vi "Dashboard Main 2022.vi"(0 "Dashboard Tab":T3(tab)) -> ()   [LabVIEW 2020]
uses:
  <vilib>/Rock Robotics/Network Tables/NT Read Number.vi
  <vilib>/Rock Robotics/Network Tables/NT Read Numeric Array.vi
  <vilib>/Rock Robotics/Network Tables/NT Read String.vi
  <vilib>/Rock Robotics/Network Tables/NT Read Boolean.vi
  <vilib>/Rock Robotics/Network Tables/NT Write Number.vi
  <vilib>/Rock Robotics/Network Tables/NT Write Boolean.vi
panel:
  out "Robot IP":string
  out "Popcorn Engaged":bool
  out "Camera Image 5":T1(plugin-control)
  out "Camera Perf":string
  in  "Camera Settings":T2={"Frame Rate"=30, "Compression"=30, "Size"=1, "DB Camera Config"=FALSE} {"Frame Rate" scale=1.0..30.0; "Compression" scale=100.0..-1.0; "Size" items=["640x480", "320x240", "160x120"]}
  in  "TCP":refnum<k5>
  out "MotorChart R":cluster{"Numeric":dbl, "Numeric":dbl}(graph)
  out "MotorChart L":cluster{"Numeric":dbl, "Numeric":dbl}(graph)
  out "MotorSliders R":cluster{"MotorSlide1":dbl, "MotorSlide2":dbl} {"MotorSlide2" scale=-1.0..1.0 scale format="%#_2e"; "MotorSlide1" scale=-1.0..1.0 scale format="%#_2e"}
  out "MotorSliders L":cluster{"MotorSlide1":dbl, "MotorSlide2":dbl} {"MotorSlide2" scale=-1.0..1.0 scale format="%#_2e"; "MotorSlide1" scale=-1.0..1.0 scale format="%#_2e"}
  out "To infinity and beyond?":string
  out "Climb Override":bool
  out "Climbing Stages":sgl(slide) scale=0.0..10.0 scale format="%#_6p"
  out "Reverse":bool
  in  "ARE YOU READY TO RUMBLE":bool
  out "Drive Mode":string
  in  "Select Auto":string(combo)="Select Autonomous ..."
  out "NT Connection":bool
  out "JS1 Z":dbl(slide) scale=-1.0..1.0 scale format="%#_2e"
  out "JS1 Graph":cluster{"X":dbl, "Y":dbl}[](graph)
  out "JS1 Buttons":T4
  out "JS2 Z":dbl(slide) scale=-1.0..1.0 scale format="%#_2e"
  out "JS2 Graph":cluster{"X":dbl, "Y":dbl}[](graph)
  out "JS2 Buttons":T4
  out "Lidar":dbl(knob) scale=0.0..10.0
  out "Wall!":bool
  out "Mode":T5(ring)=enum."Auto Disabled"
  out "Motor Output":dbl
  out "Target Shooter Speed":dbl
  out "Shooter Speed":T6(graph)
  out "Shooter Speed":dbl
  in  "Shooter Demand":dbl
  in  "Dashboard Tab 2":T7(tab)
  out "Speed Chart Left":cluster{"Numeric":dbl, "Numeric":dbl}(graph)
  out "Speed Chart Right":cluster{"Numeric":dbl, "Numeric":dbl}(graph)
  in  "Dont Question it":bool
  out "Right Speed Demand":dbl
  out "Left Speed Demand":dbl
  out "Right Speed":dbl
  out "Left Speed":dbl
  out "Deviation Threshold":dbl
  out "Filter Height":dbl
  in  "Deviation Threshold":dbl
  in  "Filter Height":dbl
  out "Current Filter":T8={"Hue"={110.0, 142.0}, "Saturation"={0.0, 209.6394230769231}, "Value"={0.0, 105.16949152542372}} {"Value" scale=0.0..255.0; "Saturation" scale=0.0..255.0; "Hue" scale=0.0..255.0 scale format="%#_3g"}
  in  "New Filter":T8={"Hue"={110.0, 142.0}, "Saturation"={0.0, 209.6394230769231}, "Value"={0.0, 105.16949152542372}} {"Value" scale=0.0..255.0; "Saturation" scale=0.0..255.0; "Hue" scale=0.0..255.0 scale format="%#_3g"}
  out "Bananas Engaged":bool
  in  "DONUT PRESS":bool
  out "Bandwidth (Mbps)":dbl
  out "FPS":dbl
  in  "Update":bool
  in  "CheckList":i32[](listbox)
  out "Tree":string(tree)
  out "Camera Image":T1(plugin-control)
  out "Background":bool
  in  "Camera Name":string(combo)="No Camera Selection"
  # "HW"
  # "Joysticks"
  # "Drive Motors"
  # "Front"
  # "Right"
  # "Left"
  # "Back"
  # "Right"
  # "Left"
  # "Speed D"
  # "Speed"
  # "DONUT PRESS"
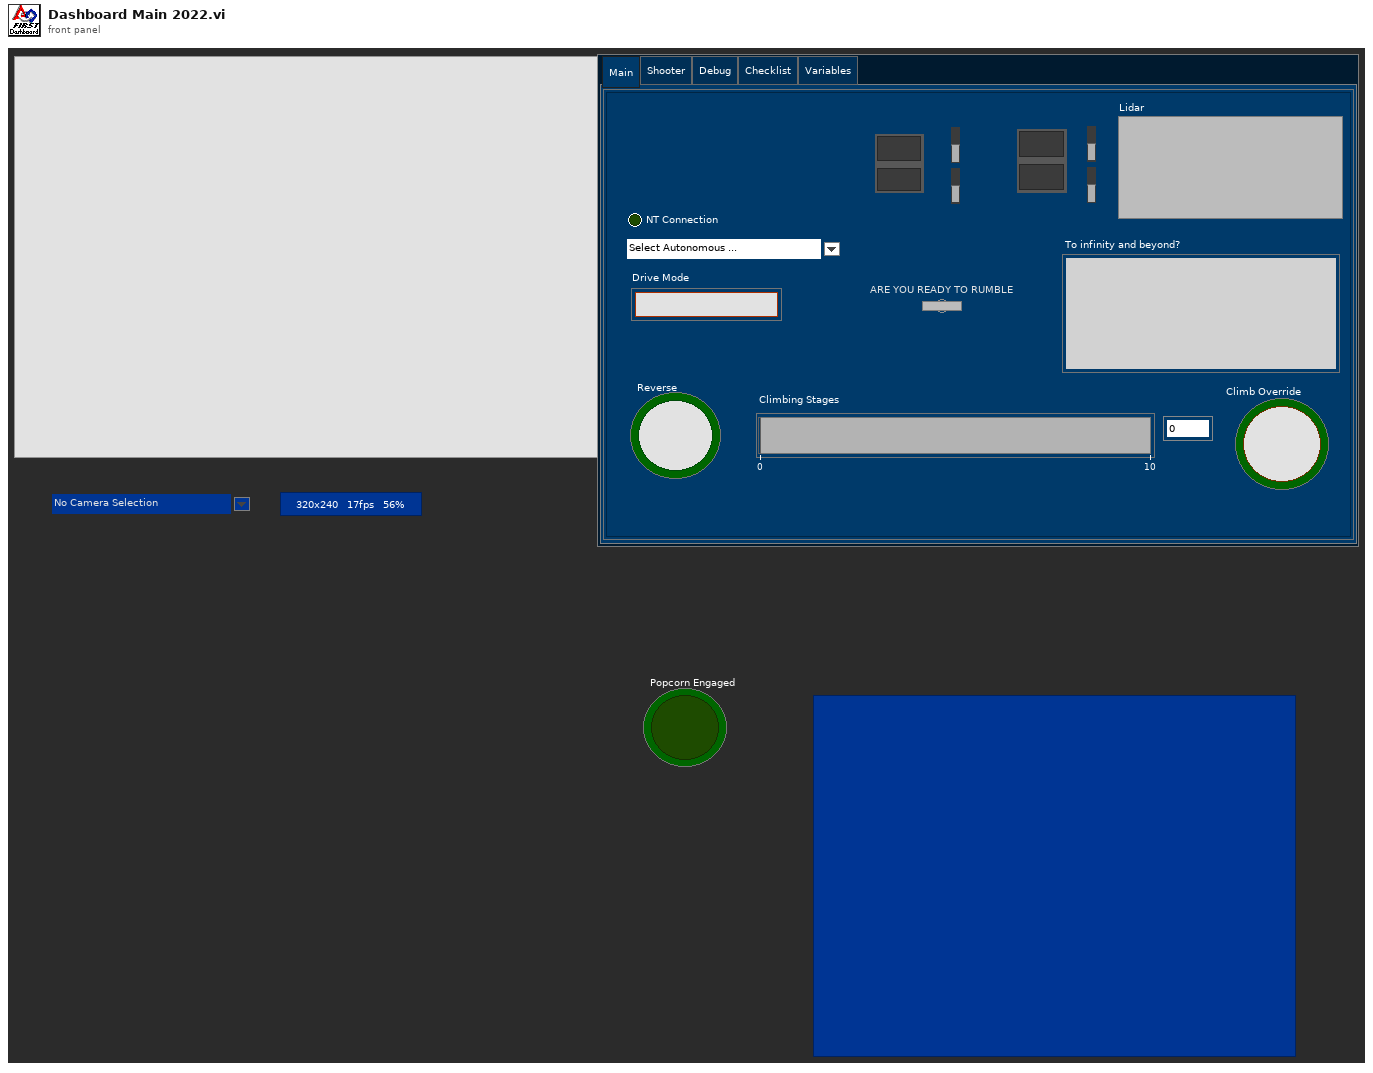
[diagram p1: front panel]
types:
  T1 = typedef "IMAQ Image.ctl" = refnum<image>
  T2 = cluster{"Frame Rate":i32, "Compression":i32, "Size":u16, "DB Camera Config":bool}
  T3 = enum32{"Main", "Shooter", "Debug", "Checklist", "Variables"}
  T4 = cluster{bool, bool, bool, bool, bool, bool, bool, bool, bool, bool, bool, bool}
  T5 = enum8{"Tele-Op Disabled", "Tele-Op Enabled", "Auto Disabled", "Auto Enabled", "Test Disabled", "Test Enabled", "Disconnected", "No Code", "E-Stop"}
  T6 = cluster{"Shooter Demand":dbl, "Numeric":dbl, "Numeric":dbl}
  T7 = enum32{"Drive Left", "Drive Right", "Table", "Camera", "Random"}
  T8 = cluster{"Hue":cluster{dbl, dbl}, "Saturation":cluster{dbl, dbl}, "Value":cluster{dbl, dbl}}
  T9 = cluster{"Save Path":path, "Interval (s)":dbl, "Keep":i32}
  T10 = typedef "Image Type" = u32
  T11 = cluster{"Camera Image":refnum<vi>, "Dashboard Tab":refnum<vi>, "Background":refnum<vi>, "Tree":refnum<vi>, "Camera Settings":refnum<vi>, "Camera Name":refnum<vi>, "Camera Perf":refnum<vi>}
  T12 = cluster{"Camera Name":string, "Camera File Name":string, "Saved DB Images Info":cluster{"Save Path":path, "Interval (s)":dbl, "Keep":i32}}
  T13 = cluster{cluster{dbl, dbl}, cluster{dbl, dbl}, cluster{dbl, dbl}}
  T14 = cluster{"Shift":bool, "Ctrl":bool, "Alt":bool, "Cmd":bool, "Opt":bool}
  T15 = cluster{"Error Strings":string, "Disable Counts":cluster{u16, u16}, "Rail Faults":cluster{u16, u16, u16}, "Robot IP":string, "DB Mode":u8, "Event Info":cluster{"Name":string, "Type":u8, "Number":u16, "Replay":u8}}
  T16 = cluster{"Storage":cluster{"Disk Free":u64, "RAM Block":u32, "RAM free":u32}, "CPU Utilization":cluster{"CPU % ISR":sgl, "CPU % Time Crit":sgl, "CPU % Timed Str":sgl, "CPU % High":sgl, "CPU % Above":sgl, "CPU % Normal":sgl, "CPU % Low":sgl}, "CAN":cluster{"% Bus Utilization":sgl, "Bus Off Cnt":u32, "TX_FIFO Full Cnt":u32, "Receive Error Cnt":u8, "Transmit Error Cnt":u8}, "HID":cluster{"HID Outputs":u32, "Rumble Low":u16, "Rumble High":u16}[]}
  T17 = cluster{"Status bits":cluster{"Test Mode":bool, "Autonomous":bool, "Enabled":bool, "Code Start":bool, "Brownout":bool, "Reserved 2":bool, "Reserved 3":bool, "E-Stop":bool}, "Code Trace":cluster{"Disabled":bool, "TeleOp":bool, "Auto":bool, "Test":bool}, "Controller Type":enum16{"unknown", "cRIO", "roboRio"}, "Code?":enum16{"unknown", "noCode", "code"}, "Battery V":dbl}
  T18 = cluster{"Control Bits":cluster{"TestMode":bool, "Autonomous":bool, "Enabled":bool, "FMS Present":bool, bool, bool, bool, "E-Stop":bool}, "Team Station ":u8, "Countdown":sgl, "Joystick Values":cluster{"Axes":dbl[], "Buttons":bool[], "POVs":i16[]}[]}
  T19 = cluster{"Axes":dbl[], "Buttons":bool[], "POVs":i16[]}[]
  T20 = cluster{"Axes":dbl[], "Buttons":bool[], "POVs":i16[]}
  T21 = cluster{"Buttons[0]":bool, "Buttons[1]":bool, "Buttons[2]":bool, "Buttons[3]":bool, "Buttons[4]":bool, "Buttons[5]":bool, "Buttons[6]":bool, "Buttons[7]":bool, "Buttons[8]":bool, "Buttons[9]":bool, "Buttons[10]":bool, "Buttons[11]":bool}
  T22 = cluster{"Shooter Demand":dbl, "value":dbl, "value":dbl}
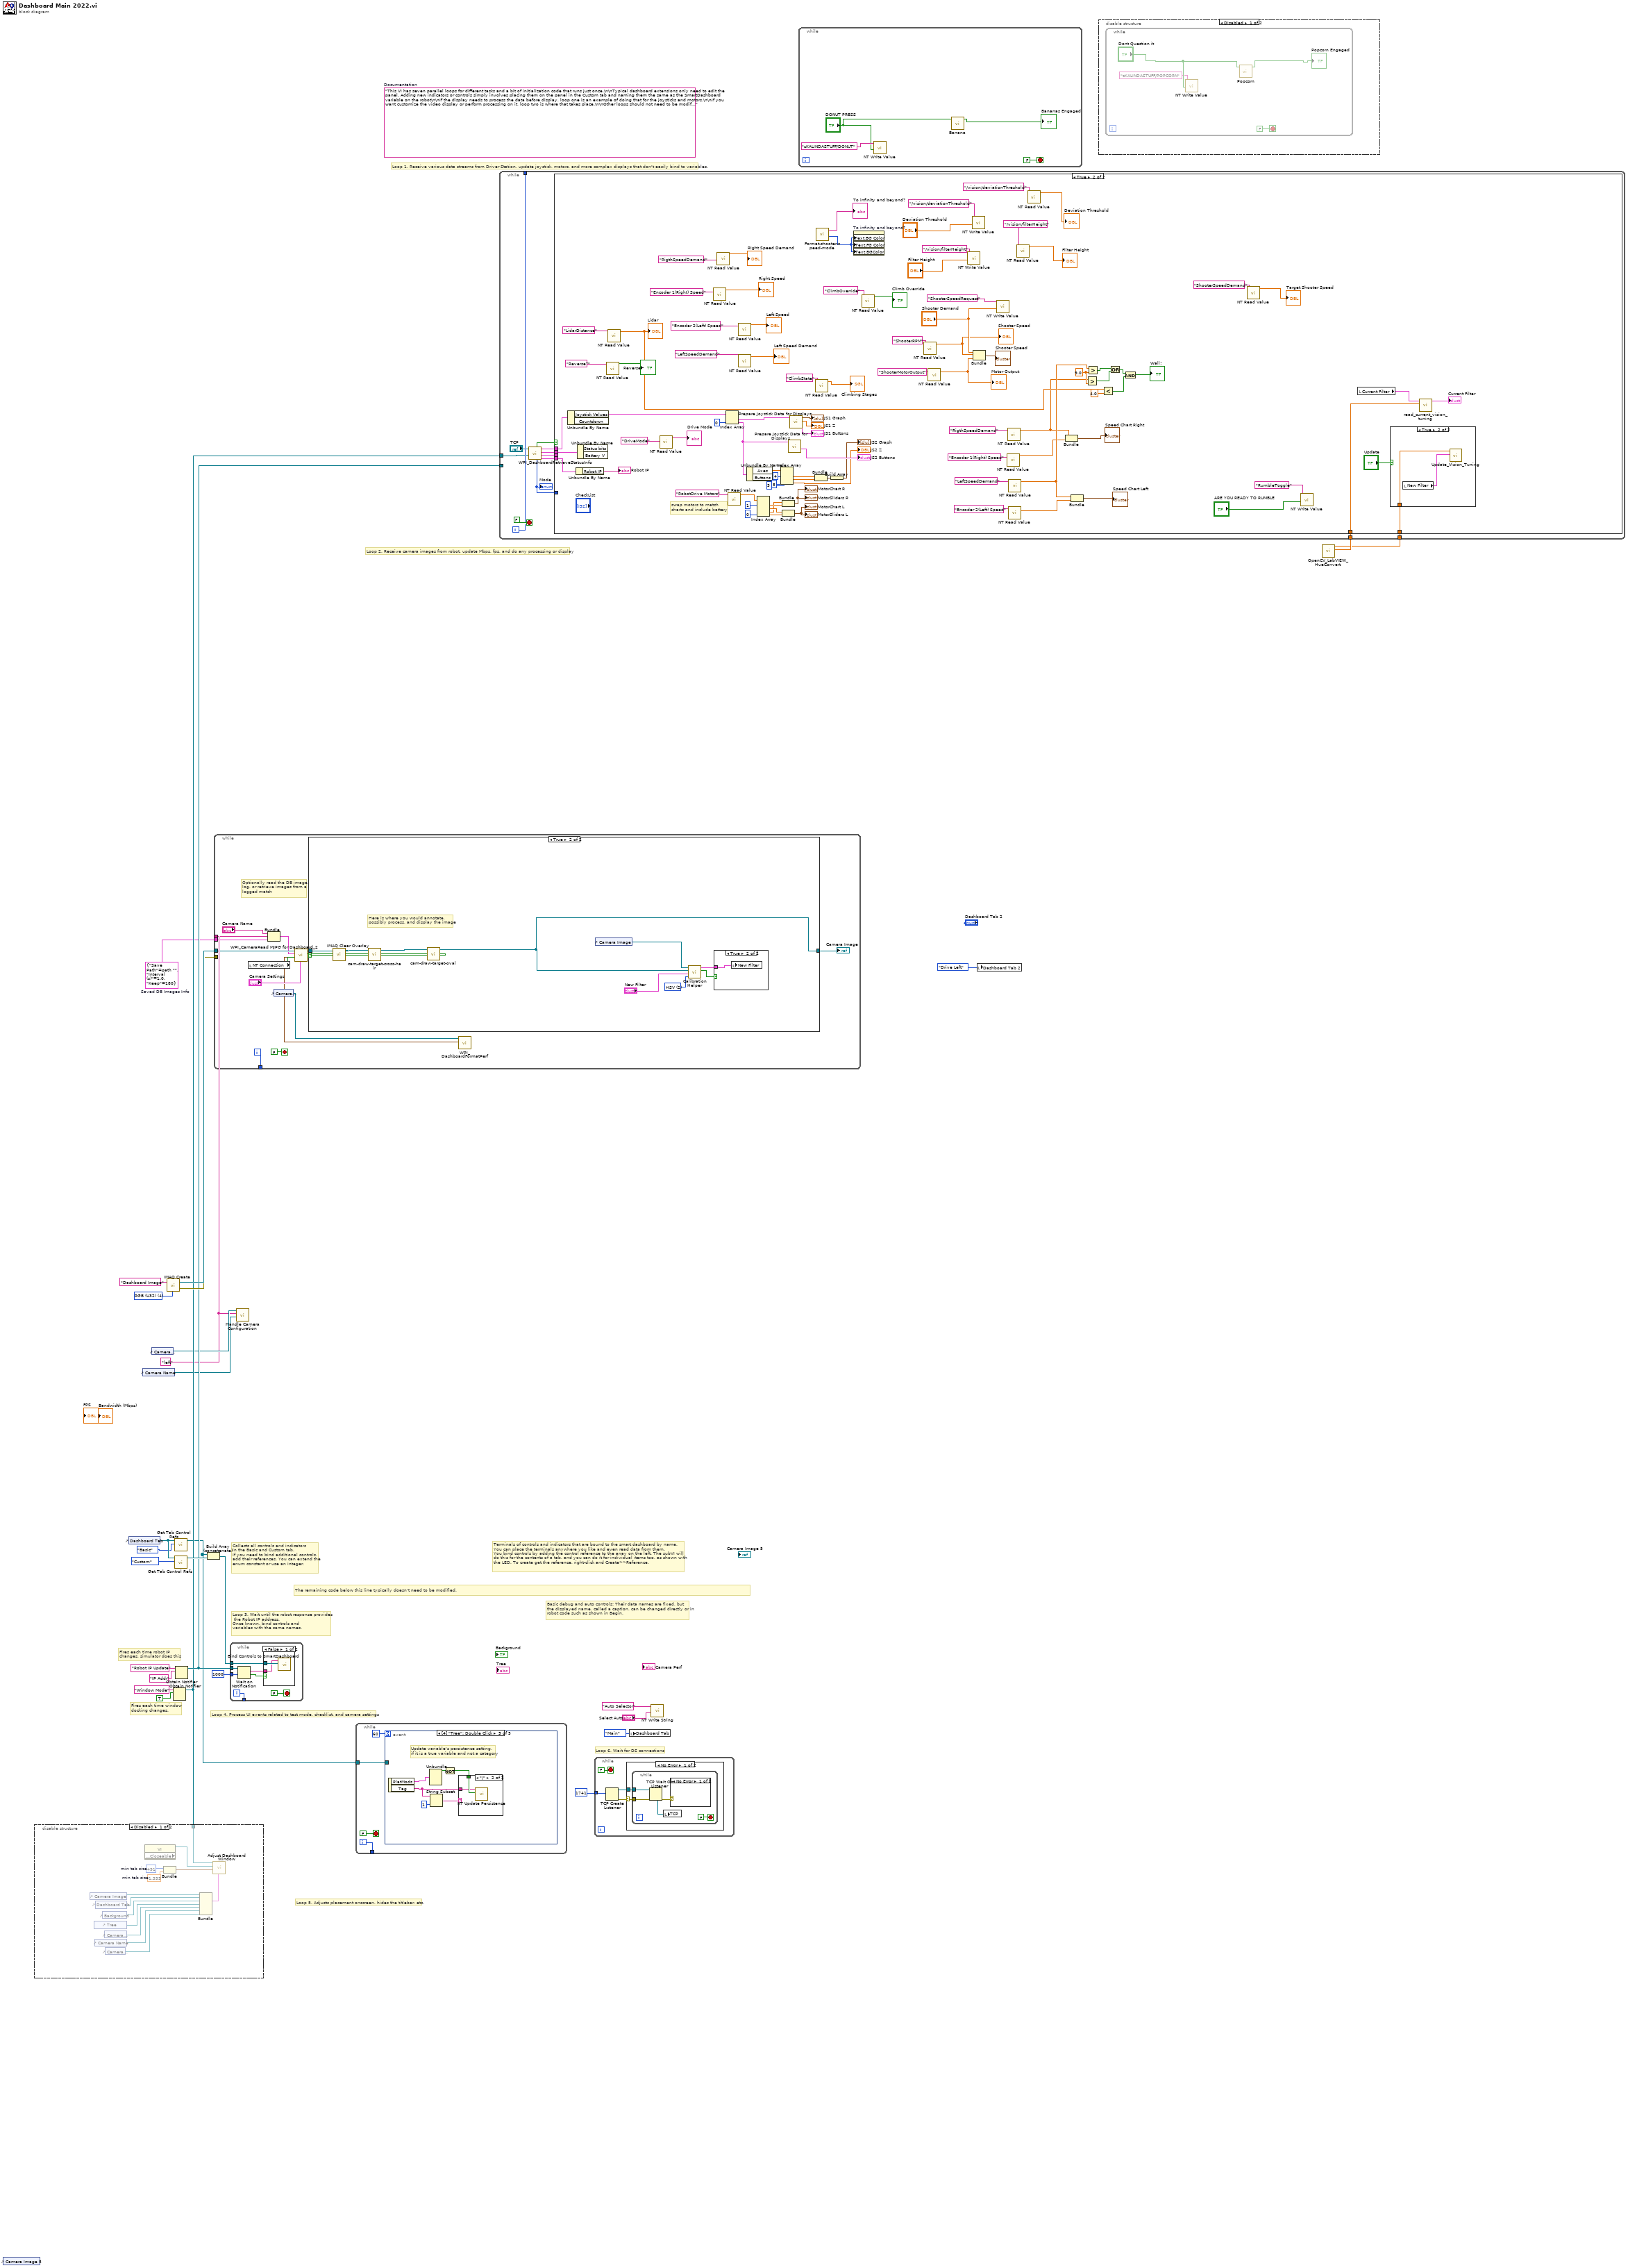
[diagram p0: block diagram]
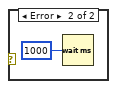
[diagram p4: hidden frame]
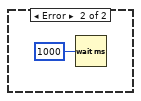
[diagram p5: hidden frame]
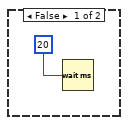
[diagram p6: hidden frame]
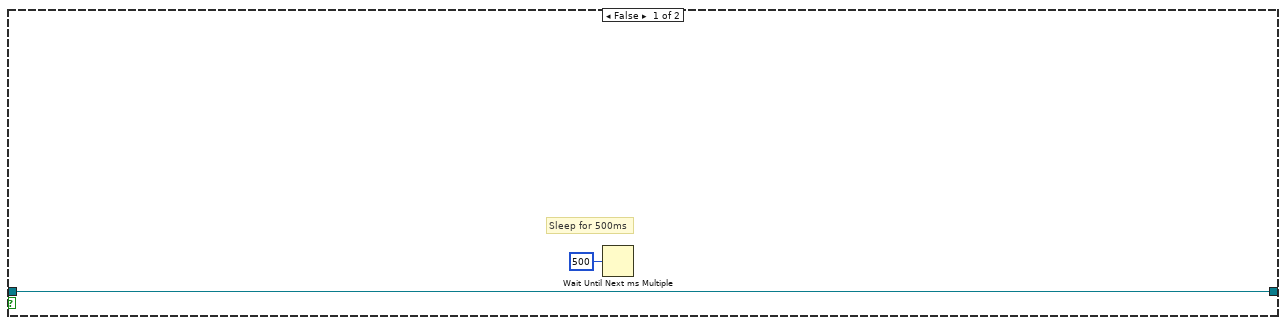
[diagram p9: hidden frame]
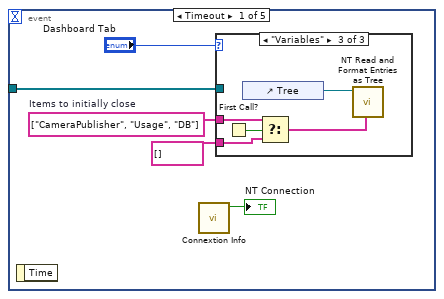
[diagram p11: hidden frame]
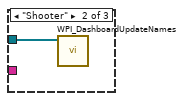
[diagram p13: hidden frame]
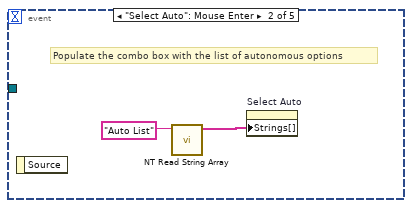
[diagram p14: hidden frame]
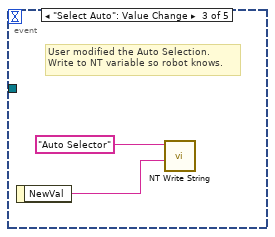
[diagram p15: hidden frame]
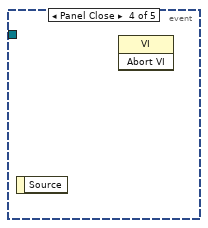
[diagram p16: hidden frame]
diagram:
  w6 = "left" ("Camera File Name")
  w5 = T9 {"Save Path"=path "", "Interval (s)"=1.0, "Keep"=180}  # Saved DB Images Info
  (unwired) "This VI has seven parallel loops for different tasks and a bit of initialization code that runs just once.\n\nTypical dashboard extensions only need to edit the panel. Adding new indicators or controls simply involves placing them on the panel in the Custom tab and naming them the same as the SmartDashboard variable on the robot\n\nIf the display needs to process the data before display, loop one is an example of doing that for the joysticks and motors.\n\nIf you want customize the video display or perform processing on it, loop two is where that takes place.\n\nOther loops should not need to be modified. They are pretty standard, and document the task they perform."  # Documentation
  w28 = T10 4 items=["Grayscale (U8)", "Grayscale (I16)", "Grayscale (SGL)", "Complex (CSG)", "RGB (U32)", "HSL (U32)", "RGB (U64)"] ("Image Type")
  # "Loop 5. Adjusts placement onscreen, hides the titlebar, etc."
  # "Loop 6. Wait for DS connections"
  # "Basic debug and auto controls: Their data names are fixed, but\nthe displayed name, called a caption, can be changed directly or in\nrobot code such as shown in Begin."
  # "Fires each time robot IP\nchanges, simulator does this"
  # "Fires each time window\ndocking changes."
  # "Collects all controls and indicators\nin the Basic and Custom tab.\nIf you need to bind additional controls,\nadd their references. You can extend the\nenum constant or use an integer."
  # "The remaining code below this line typically doesn't need to be modified."
  # "Loop 4. Process UI events related to test mode, checklist, and camera settings"
  # "Terminals of controls and indicators that are bound to the smart dashboard by name.\nYou can place the terminals anywhere you like and even read data from them.\nYou bind controls by adding the control reference to the array on the left. The subVI will\ndo this for the contents of a tab, and you can do it for individual items too, as shown with\nthe LED. To create get the reference, right-click and Create>>Reference."
  # "Loop 3. Wait until the robot response provides\n the Robot IP address.\nOnce known, bind controls and\nvariables with the same names."
  # "Loop 1. Receive various data streams from Driver Station, update joystick, motors, and more complex displays that don't easily bind to variables."
  # "Loop 2. Receive camera images from robot, update Mbps, fps, and do any processing or display"
  n1 = control-ref of="Camera Image 5"() -> ()  [unwired: 1 out]
  n2 = control-ref of="Dashboard Tab"() -> (w19:refnum<vi>)
  n3 = control-ref of="Camera Name"() -> (w12:refnum<vi>)
  n4 = control-ref of="Camera Settings"() -> (w13:refnum<vi>)
  n5 = call "IMAQ Create"("Image Name"="Dashboard Image", "Image Type"=w28) -> ("New Image"=w26:T1, "error out"=w25:errorcluster)  [unwired: 2 in, 1 out]
  n6 = Obtain Notifier(name (unnamed)="Window Mode", notification data type=TRUE) -> (notifier out=w15:refnum<notifier>)  [unwired: 2 in, 2 out]
  n7 = disable-structure shown="Disabled" {
    disable-tunnel: w15 -> [w33 _]
    frame Disabled {
      w38 = 491  # min tab size
      w37 = 1.333  # min tab size
      n8 = control-ref of="Camera Image"() -> (w40:refnum<vi>)
      n9 = control-ref of="Tree"() -> (w32:refnum<vi>)
      n10 = control-ref of="Camera Name"() -> (w30:refnum<vi>)
      n11 = control-ref of="Dashboard Tab"() -> (w39:refnum<vi>)
      n12 = control-ref of="Background"() -> (w35:refnum<vi>)
      n13 = control-ref of="Camera Settings"() -> (w31:refnum<vi>)
      n14 = control-ref of="Camera Perf"() -> (w29:refnum<vi>)
      n15 = property class="VI" props=["Front Panel.Closeable"]() -> (reference out=w41:refnum<vi>)  [unwired: 2 in, 2 out]
      n16 = Bundle("min tab size"=w38, "min tab size"=w37) -> (w36:cluster{"min tab size":i32, "min tab size":dbl})  [unwired: 1 in]
      n17 = Bundle("Camera Image"=w40, "Dashboard Tab"=w39, "Background"=w35, "Tree"=w32, "Camera Settings"=w31, "Camera Name"=w30, "Camera Perf"=w29) -> (w34:T11)  [unwired: 1 in]
      n18 = call "Adjust Dashboard Window.vi"("Sizing Refnums"=w34, "Size Constraints"=w36, "VI"=w41, "WIn Mode"=w33) -> ()  [unwired: 8 in]
    }
    frame Enabled {
    }
  }
  n19 = call <vilib>:"Get Tab Control Refs.vi"("Page Index"=enum32{"Drive", "Basic", "Custom", "Variables"}."Basic" ("Dashboard Tab"), "TabControl in"=w19) -> ("ControlsOnPage"=w11:refnum<vi>[])  [unwired: 9 in]
  n20 = call <vilib>:"Get Tab Control Refs.vi"("Page Index"=enum32{"Drive", "Basic", "Custom", "Variables"}."Custom" ("Dashboard Tab"), "TabControl in"=w19) -> ("ControlsOnPage"=w18:refnum<vi>[])  [unwired: 9 in]
  n21 = Obtain Notifier(name (unnamed)="Robot IP Update", notification data type="IP Addr" ("name (unnamed)")) -> (notifier out=w16:refnum<notifier>)  [unwired: 2 in, 2 out]
  n22 = Build Array (concatenate)(w11, w18) -> (w17:refnum<vi>[])
  n23 = while {
    tunnel: w26 -> [w53]
    tunnel: w25 -> [_]
    tunnel: [w54] -> _
    tunnel: w5 -> [w47]
    tunnel: w6 -> [w45]
    i -> [w54]
    stop <- FALSE stop-if-true
    # "Optionally read the DB image,\nlog, or retrieve images from a\nlogged match"
    n24 = local read "NT Connection"() -> (w48:bool)
    n25 = Bundle("Camera Name"="Camera Name", "Camera File Name"=w45, "Saved DB Images Info"=w47) -> (w46:T12)  [unwired: 1 in]
    n26 = control-ref of="Camera Perf"() -> (w43:refnum<vi>)
    n27 = call <vilib>:"WPI_CameraRead MJPG for Dashboard_2.vi"("Camera Settings"="Camera Settings", "NT Connection"=w48, "Capture Info"=w46, "Image in"=w53) -> ("perf info"=w44:cluster{"Bandwidth (Mbps)":dbl, "fps":dbl}, "Active"=w51:bool, "Image\\ out"=w52:T1)  [unwired: 5 in]
    n28 = case shown="True" w51 {
      tunnel: w52 -> [w56 w66]
      tunnel: [w56 w58] -> w49
      frame False {
        # "Sleep for 500ms"
        n29 = Wait Until Next ms Multiple(millisecond multiple=u32 500) -> ()  [unwired: 1 out]
      }
      frame True {
        w62 = u16 2 items=["RGB", "HSL", "HSV", "HSI", "CIE L*a*b*", "CIE XYZ"] ("Color Mode")
        # "Here is where you would annotate,\npossibly process, and display the image"
        n30 = call "IMAQ Clear Overlay"("Image"=w66) -> ("Image Out"=w60:T1)  [unwired: 2 in, 8 out]
        n31 = call "cam-draw-target-cross-hair.vi"("Refnum in"=w60) -> ("Refnum out"=w59:T1)  [unwired: 10 in]
        n32 = call "cam-draw-target-oval.vi"("Refnum in"=w59) -> ("Refnum out"=w58:T1)  [unwired: 10 in]
        n33 = control-ref of="Camera Image"() -> (w61:refnum<vi>)
        n34 = call "Calibration Helper.vi"("Color Mode"=w62, "Color Components"="New Filter", "Image"=w58, "Image Ctl Refnum"=w61) -> ("Changed"=w64:bool, "output color"=w63:T13)  [unwired: 6 in]
        n35 = case shown="True" w64 {
          tunnel: w63 -> [_ w67]
          frame False {
          }
          frame True {
            n36 = local write "New Filter"(w67) -> ()
          }
        }
      }
    }
    "Camera Image" <- w49
    n37 = call <vilib>:"WPI_DashboardFormatPerf.vi"("Performance"=w44, "String in"=w43) -> ()  [unwired: 10 in]
  }
  n38 = while {
    tunnel: w17 -> [w74]
    tunnel: w16 -> [w72]
    tunnel: [w70] -> _
    tunnel: u32 1000 ("milliseconds to wait") -> [w69]
    i -> [w70]
    stop <- FALSE stop-if-true
    n39 = Wait on Notification(notifier=w72, timeout in ms (-1)=w69) -> (notification=w71:string, timed out?=w68:bool)  [unwired: 2 in, 2 out]
    n40 = case shown="False" w68 {
      tunnel: w74 -> [w76 _]
      tunnel: w71 -> [w75 _]
      frame False {
        n41 = call <vilib>:"Bind Controls to SmartDashboard.vi"("Bound Control Refs"=w76, "Server IP Address"=w75) -> ()  [unwired: 10 in]
      }
      frame True {
      }
    }
  }
  n42 = call "Handle Camera Configuration.vi"("CameraNameRef"=w12, "Display Name"=w6, "ClusterRef"=w13) -> ()  [unwired: 9 in]
  n43 = while {
    tunnel: [w78] -> _
    tunnel: w11 -> [w77]
    i -> [w78]
    stop <- FALSE stop-if-true
    n44 = event shown="[4] \"Tree\": Double Click" {
      selector: _ -> [_ _ _ _ _]
      dyn-events: _ -> [_ _ _ _ _]
      timeout: u32 60 ("milliseconds to wait") -> [_ _ _ _ _]
      tunnel: w77 -> [w83 _ _ _ _]
      event Timeout {
        w82 = string[] ["CameraPublisher", "Usage", "DB"]  # Items to initially close
        n45 = event-data() -> ()  [unwired: 1 in, 1 out]
        n46 = call <vilib>:"Connextion Info.vi"() -> ("Connected"=→"NT Connection":bool)  [unwired: 10 in, 1 out]
        n47 = case shown="\"Variables\"" "Dashboard Tab" {
          tunnel: w83 -> [_ w86 _]
          tunnel: w82 -> [_ _ w89]
          tunnel: string[] [] -> [_ _ w88]
          frame "Debug", Default {
          }
          frame "Shooter" {
            n48 = call <vilib>:"WPI_DashboardUpdateNames.vi"("Controls on Tab"=w86) -> ()  [unwired: 11 in]
          }
          frame "Variables" {
            n49 = First Call?() -> (First Call?: T/F=w90:bool)
            n50 = control-ref of="Tree"() -> (w91:refnum<vi>)
            n51 = Select(t=w89, s=w90, f=w88) -> (s? t:f=w87:string[])
            n52 = call <vilib>:"NT Read and Format Entries as Tree.vi"("Tags to  Close"=w87, "Tree Refnum"=w91) -> ()  [unwired: 8 in, 2 out]
          }
        }
      }
      event "Select Auto": Mouse Enter {
        # "Populate the combo box with the list of autonomous options"
        n53 = event-data() -> ()  [unwired: 1 in, 1 out]
        n54 = call <vilib>:"NT Read String Array.vi"("name"="Auto List" ("Name")) -> ("value"=w92:string[])  [unwired: 8 in, 2 out]
        n55 = property on="Select Auto" class="CmbBox"("Strings[]"=w92) -> ()  [unwired: 2 in, 2 out]
      }
      event "Select Auto": Value Change {
        # "User modified the Auto Selection.\nWrite to NT variable so robot knows."
        n56 = event-data() -> ("NewVal"=w94:string)  [unwired: 1 in]
        n57 = call <vilib>:"NT Write String.vi"("value"=w94, "name"="Auto Selector" ("Name")) -> ()  [unwired: 9 in, 1 out]
      }
      event Panel Close {
        n58 = event-data() -> ()  [unwired: 1 in, 1 out]
        n59 = invoke class="VI" method="Abort VI"() -> ()  [unwired: 3 in, 3 out]
      }
      event "Tree": Double Click {
        # "Update variable's persistence setting,\nif it is a true variable and not a category"
        n60 = event-data() -> ("PlatMods"=w97:T14, "Tag"=w96:string)  [unwired: 1 in]
        n61 = Unbundle(w97) -> ("Shift"=w101:bool)  [unwired: 4 out]
        n62 = String Subset(string=w96, length (rest)=1 ("length (rest)")) -> (substring=w98:string)  [unwired: 1 in]
        n63 = Not(x=w101) -> (.not. x?=w100:bool)
        n64 = case shown="\"/\"" w98 {
          tunnel: w100 -> [_ w103]
          tunnel: w96 -> [_ w102]
          frame Default {
          }
          frame "/" {
            n65 = call <vilib>:"NT Update Persistence.vi"("Persistence"=w103, "Name"=w102) -> ()  [unwired: 9 in, 1 out]
          }
        }
      }
    }
  }
  n66 = while {
    tunnel: u16 1741 ("timeout ms (25000)") -> [w105]
    stop <- FALSE stop-if-true
    n67 = TCP Create Listener(10:w105) -> (0:w104:errorcluster, 3:w106:refnum<k5>)  [unwired: 4 in, 1 out]
    n68 = case shown="No Error" w104 {
      selector: w104 -> [w108 _]
      tunnel: w106 -> [w109 _]
      frame No Error {
        n69 = while {
          tunnel: w109 -> [w112]
          tunnel: w108 -> [w111]
          stop <- FALSE stop-if-true
          n70 = TCP Wait On Listener(8:w111, 11:w112) -> (0:w113:errorcluster, 4:w114:refnum<k5>)  [unwired: 2 in, 3 out]
          n71 = local write "TCP"(w114) -> ()
          n72 = case shown="No Error" w113 {
            frame No Error {
            }
            frame Error {
              n73 = Wait (ms)(milliseconds to wait=u32 1000) -> ()  [unwired: 1 out]
            }
          }
        }
      }
      frame Error {
        n74 = Wait (ms)(milliseconds to wait=u32 1000) -> ()  [unwired: 1 out]
      }
    }
  }
  n75 = local write "Dashboard Tab"(T3."Main" ("Dashboard Tab")) -> ()
  n76 = call <vilib>:"NT Write String.vi"("value"="Select Auto", "name"="Auto Selector" ("Name")) -> ()  [unwired: 9 in, 1 out]
  n77 = while {
    stop <- FALSE stop-if-true
    n78 = call-poly <vilib>:"NT Write Value.vi"("value"="DONUT PRESS", "name"="zKALINDASTUFF/DONUT" ("Name")) -> ()  [unwired: 9 in, 1 out]
    n79 = call "Banana.vi"("Boolean"="DONUT PRESS") -> ("Boolean 2"=→"Bananas Engaged":bool)  [unwired: 10 in]
  }
  n80 = local write "Dashboard Tab 2"(T7."Drive Left" ("Dashboard Tab")) -> ()
  n81 = disable-structure shown="Disabled" {
    frame Disabled {
      n82 = while {
        stop <- FALSE stop-if-true
        n83 = call-poly <vilib>:"NT Write Value.vi"("value"="Dont Question it", "name"="zKALINDASTUFF/POPCORN" ("Name")) -> ()  [unwired: 9 in, 1 out]
        n84 = call "Popcorn.vi"("Boolean"="Dont Question it") -> ("Boolean 2"=→"Popcorn Engaged":bool)  [unwired: 10 in]
      }
    }
    frame Enabled {
    }
  }
  n85 = call "OpenCV_LabVIEW_HueConvert.vi"() -> ("OpenCV to LV"=w3:dbl, "LV to OpenCV"=w2:dbl)  [unwired: 10 in]
  n86 = while {
    tunnel: [w135] -> _
    tunnel: w16 -> [_]
    tunnel: w15 -> [w127]
    tunnel: w3 -> [w126]
    tunnel: w2 -> [w125]
    i -> [w135]
    stop <- FALSE stop-if-true
    n87 = call <vilib>:"WPI_DashboardRetrieveStatusInfo.vi"("Window Mode Notifier"=w127, "TCP Cnx"="TCP") -> ("Power and Errors"=w130:T15, "Robot Metrics"=w133:T16, "Status Info"=w134:T17, "Control Info"=w131:T18, "Robot Mode"=w129:T5, "Process?"=w132:bool)  [unwired: 4 in]
    "Mode" <- w129
    n88 = case shown="True" w132 {
      tunnel: w134 -> [_ w229]
      tunnel: w133 -> [_ _]
      tunnel: w131 -> [_ w228]
      tunnel: w130 -> [_ w227]
      tunnel: w129 -> [_ _]
      tunnel: w126 -> [_ w183]
      tunnel: w125 -> [_ w181]
      frame False {
        n89 = Wait (ms)(milliseconds to wait=u32 20) -> ()  [unwired: 1 out]
      }
      frame True {
        w157 = 9.0 ("y")
        # "swap motors to match\ncharts and include battery"
        n90 = Unbundle By Name(w228) -> ("Joystick Values"=w218:T19)  [unwired: 1 out]
        n91 = Unbundle By Name(w227) -> ("Robot IP"=→"Robot IP":string)
        n92 = Unbundle By Name(w229) -> ()  [unwired: 2 out]
        n93 = call-poly <vilib>:"NT Read Value.vi"("name"="Reverse?") -> ("value"=→"Reverse":bool)  [unwired: 8 in, 2 out]
        n94 = call-poly <vilib>:"NT Read Value.vi"("name"="LidarDistance") -> ("value"=w154:dbl)  [unwired: 8 in, 2 out]
        "Lidar" <- w154
        n95 = call-poly <vilib>:"NT Read Value.vi"("name"="DriveMode" ("Name")) -> ("value"=→"Drive Mode":string)  [unwired: 8 in, 2 out]
        n96 = call-poly <vilib>:"NT Read Value.vi"("name"="Encoder 1(Right) Speed" ("Name")) -> ("value"=→"Right Speed":dbl)  [unwired: 8 in, 2 out]
        n97 = call-poly <vilib>:"NT Read Value.vi"("name"="RigthSpeedDemand" ("Name")) -> ("value"=→"Right Speed Demand":dbl)  [unwired: 8 in, 2 out]
        n98 = Index Array(array=w218, index #2=0 ("index")) -> (element #1=w217:T20, element #2=w168:T20)  [unwired: 1 in]
        n99 = call-poly <vilib>:"NT Read Value.vi"("name"="RobotDrive Motors" ("Name")) -> ("value"=w211:dbl[])  [unwired: 8 in, 2 out]
        n100 = call-poly <vilib>:"NT Read Value.vi"("name"="Encoder 2(Left) Speed" ("Name")) -> ("value"=→"Left Speed":dbl)  [unwired: 8 in, 2 out]
        n101 = call-poly <vilib>:"NT Read Value.vi"("name"="LeftSpeedDemand" ("Name")) -> ("value"=→"Left Speed Demand":dbl)  [unwired: 8 in, 2 out]
        n102 = Unbundle By Name(w168) -> ("Axes"=w172:dbl[])  [unwired: 1 out]
        n103 = Index Array(array=w211, index #1=1, index #4=0) -> (element #1=w222:dbl, element #2=w223:dbl, element #3=w221:dbl, element #4=w226:dbl)  [unwired: 2 in]
        n104 = Index Array(array=w172, index #1=4 ("index"), index #2=5 ("index"), index #3=3 ("index")) -> (element #1=w170:dbl, element #2=w169:dbl, element #3=→"JS2 Z":dbl)
        n105 = Bundle("Numeric"=w221, "Numeric"=w222) -> (→"MotorChart R" →"MotorSliders R":cluster{"Numeric":dbl, "Numeric":dbl})  [unwired: 1 in]
        n106 = Bundle("Numeric"=w223, "Numeric"=w226) -> (→"MotorChart L" →"MotorSliders L":cluster{"Numeric":dbl, "Numeric":dbl})  [unwired: 1 in]
        n107 = call "Prepare Joystick Data for Displays.vi"("Joystick Values"=w168) -> ("Buttons"=→"JS2 Buttons":T21)  [unwired: 8 in, 2 out]
        n108 = call "Prepare Joystick Data for Displays.vi"("Joystick Values"=w217) -> ("Buttons"=→"JS1 Buttons":T21, "Z Axis"=→"JS1 Z":dbl, "Cartesian Data"=→"JS1 Graph":cluster{"X axis":dbl, "X axis":dbl}[])  [unwired: 8 in]
        n109 = Bundle("X axis"=w170, "X axis"=w169) -> (w171:cluster{"X axis":dbl, "X axis":dbl})  [unwired: 1 in]
        n110 = call-poly <vilib>:"NT Read Value.vi"("name"="ClimbState" ("Name")) -> ("value"=→"Climbing Stages":dbl)  [unwired: 8 in, 2 out]
        n111 = call "Format-shooter-speed-mode.vi"() -> ("Shooter Speed Mode Color"=w138:u32, "Shooter Speed Mode Text"=→"To infinity and beyond?":string)  [unwired: 10 in]
        n112 = Build Array(w171) -> (→"JS2 Graph":cluster{"X axis":dbl, "X axis":dbl}[])
        n113 = property on="To infinity and beyond?" class="Str"("Text.BG Color"=w138, "Text.FG Color"=w138, "Text.BGColor"=w138) -> ()  [unwired: 2 in, 2 out]
        n114 = call-poly <vilib>:"NT Read Value.vi"("name"="ClimbOverride" ("Name")) -> ("value"=→"Climb Override":bool)  [unwired: 8 in, 2 out]
        n115 = call-poly <vilib>:"NT Read Value.vi"("name"="ShooterRPM" ("Name")) -> ("value"=w185:dbl)  [unwired: 8 in, 2 out]
        "Shooter Speed" <- w185
        n116 = call-poly <vilib>:"NT Read Value.vi"("name"="ShooterMotorOutput" ("Name")) -> ("value"=w150:dbl)  [unwired: 8 in, 2 out]
        "Motor Output" <- w150
        n117 = call-poly <vilib>:"NT Write Value.vi"("value"="Filter Height", "name"="/vision/filterHeight" ("Name")) -> ()  [unwired: 9 in, 1 out]
        n118 = call-poly <vilib>:"NT Write Value.vi"("value"="Deviation Threshold", "name"="/vision/deviationThreshold" ("Name")) -> ()  [unwired: 9 in, 1 out]
        n119 = Bundle("Shooter Demand"="Shooter Demand", "value"=w185, "value"=w150) -> (→"Shooter Speed":T22)  [unwired: 1 in]
        n120 = call-poly <vilib>:"NT Write Value.vi"("value"="Shooter Demand", "name"="ShooterSpeedRequest" ("Name")) -> ()  [unwired: 9 in, 1 out]
        n121 = call-poly <vilib>:"NT Read Value.vi"("name"="Encoder 1(Right) Speed" ("Name")) -> ("value"=w148:dbl)  [unwired: 8 in, 2 out]
        n122 = call-poly <vilib>:"NT Read Value.vi"("name"="RigthSpeedDemand" ("Name")) -> ("value"=w149:dbl)  [unwired: 8 in, 2 out]
        n123 = call-poly <vilib>:"NT Read Value.vi"("name"="Encoder 2(Left) Speed" ("Name")) -> ("value"=w203:dbl)  [unwired: 8 in, 2 out]
        n124 = call-poly <vilib>:"NT Read Value.vi"("name"="LeftSpeedDemand" ("Name")) -> ("value"=w156:dbl)  [unwired: 8 in, 2 out]
        n125 = call-poly <vilib>:"NT Read Value.vi"("name"="/vision/filterHeight" ("Name")) -> ("value"=→"Filter Height":dbl)  [unwired: 8 in, 2 out]
        n126 = call-poly <vilib>:"NT Read Value.vi"("name"="/vision/deviationThreshold" ("Name")) -> ("value"=→"Deviation Threshold":dbl)  [unwired: 8 in, 2 out]
        n127 = Bundle("value"=w149, "value"=w148) -> (→"Speed Chart Right":cluster{"value":dbl, "value":dbl})  [unwired: 1 in]
        n128 = Bundle("value"=w156, "value"=w203) -> (→"Speed Chart Left":cluster{"value":dbl, "value":dbl})  [unwired: 1 in]
        n129 = Greater?(x=w149, y=w157) -> (0:w161:bool)
        n130 = Greater?(x=w156, y=w157) -> (0:w162:bool)
        n131 = Less?(x=w154, y=4.0) -> (x < y?=w160:bool)
        n132 = Or(x=w162, y=w161) -> (x .or. y?=w159:bool)
        n133 = And(x=w159, y=w160) -> (x .and. y?=→"Wall!":bool)
        n134 = call-poly <vilib>:"NT Read Value.vi"("name"="ShooterSpeedDemand" ("Name")) -> ("value"=→"Target Shooter Speed":dbl)  [unwired: 8 in, 2 out]
        n135 = call-poly <vilib>:"NT Write Value.vi"("value"="ARE YOU READY TO RUMBLE", "name"="RumbleToggle" ("Name")) -> ()  [unwired: 9 in, 1 out]
        n136 = local read "Current Filter"() -> (w180:T8)
        n137 = case shown="True" "Update" {
          tunnel: w181 -> [_ w230]
          frame False {
          }
          frame True {
            n138 = local read "New Filter"() -> (w231:T8)
            n139 = call "Update_Vision_Tuning.vi"("New Filter"=w231, "LV to OpenCV"=w230) -> ()  [unwired: 10 in]
          }
        }
        n140 = call "read_current_vision_tuning.vi"("OpenCV to LV"=w183, "Current Filter in"=w180) -> ("Current Filter out"=→"Current Filter":T8)  [unwired: 9 in]
      }
    }
  }
